vi "2D Histogram or PDF, PN.vi"(0 "Nbins U":i32, 1 "Nbins V":i32, 2 "Mean shift":bool, 3 "Umean":dbl, 4 "Vmean":dbl, 5 "Umax":dbl, 6 "No. of blocks":i32, 7 "Umin":dbl, 8 "PDF":bool, 9 "Interactive graph":bool, 10 "V":dbl[](array[numeric]), 11 "Vmax":dbl, 12 "U":dbl[](array[numeric]), 13 "Vmin":dbl) -> (14 "2D histogram or PDF":dbl[][](array[numeric]), 16 "U bin centre vals.":dbl[](array[numeric]), 17 "V bin centre vals.":dbl[](array[numeric]), 18 "UbinWidth":dbl, 19 "VbinWidth":dbl)   [LabVIEW 2011]
panel:
  in  "stop":bool
  in  "2D histogram or pdf":refnum<k7>(container)
  in  "show projections only":bool
  in  "yz projection":bool=TRUE
  in  "xz projection":bool=TRUE
  in  "xy projection":bool=TRUE
  in  "plot style":i32(ring)=9 items=["cwLine"=1, "cwPoint"=2, "cwLinePoint"=3, "cwHiddenLine"=4, "cwSurface"=5, "cwSurfaceLine"=6, "cwSurfaceNormal"=7, "cwContourLine"=8, "cwSurfaceContour"=9]
  in  "transparency":i32(knob)=40 scale=0.0..100.0
  # "N.B. The values of Umax, Umin, Vmax, Vmin, Umean, Vmean MUST be those of the ENTIRE dataset (i.e. all blocks) otherwise this routine will be inconsistent and therefore tell lies to you!!\n\nTo use this vi in a block by block manner, take note of the above and then simply add the resulting joint histogram / pdf array from each block as you go."
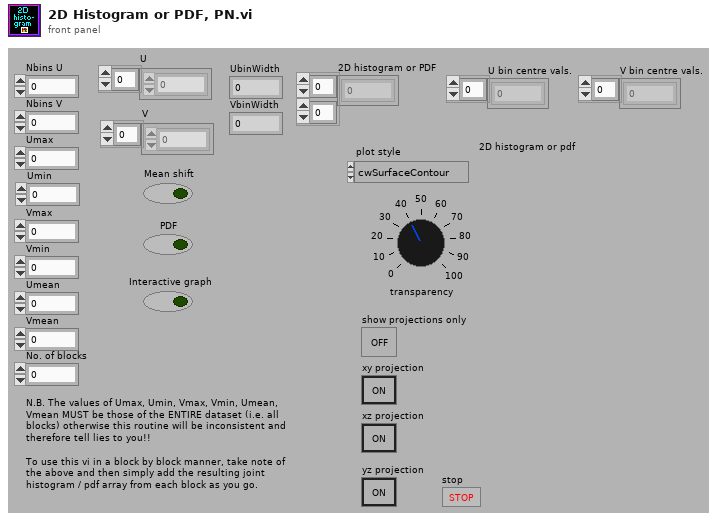
[diagram p1: front panel]
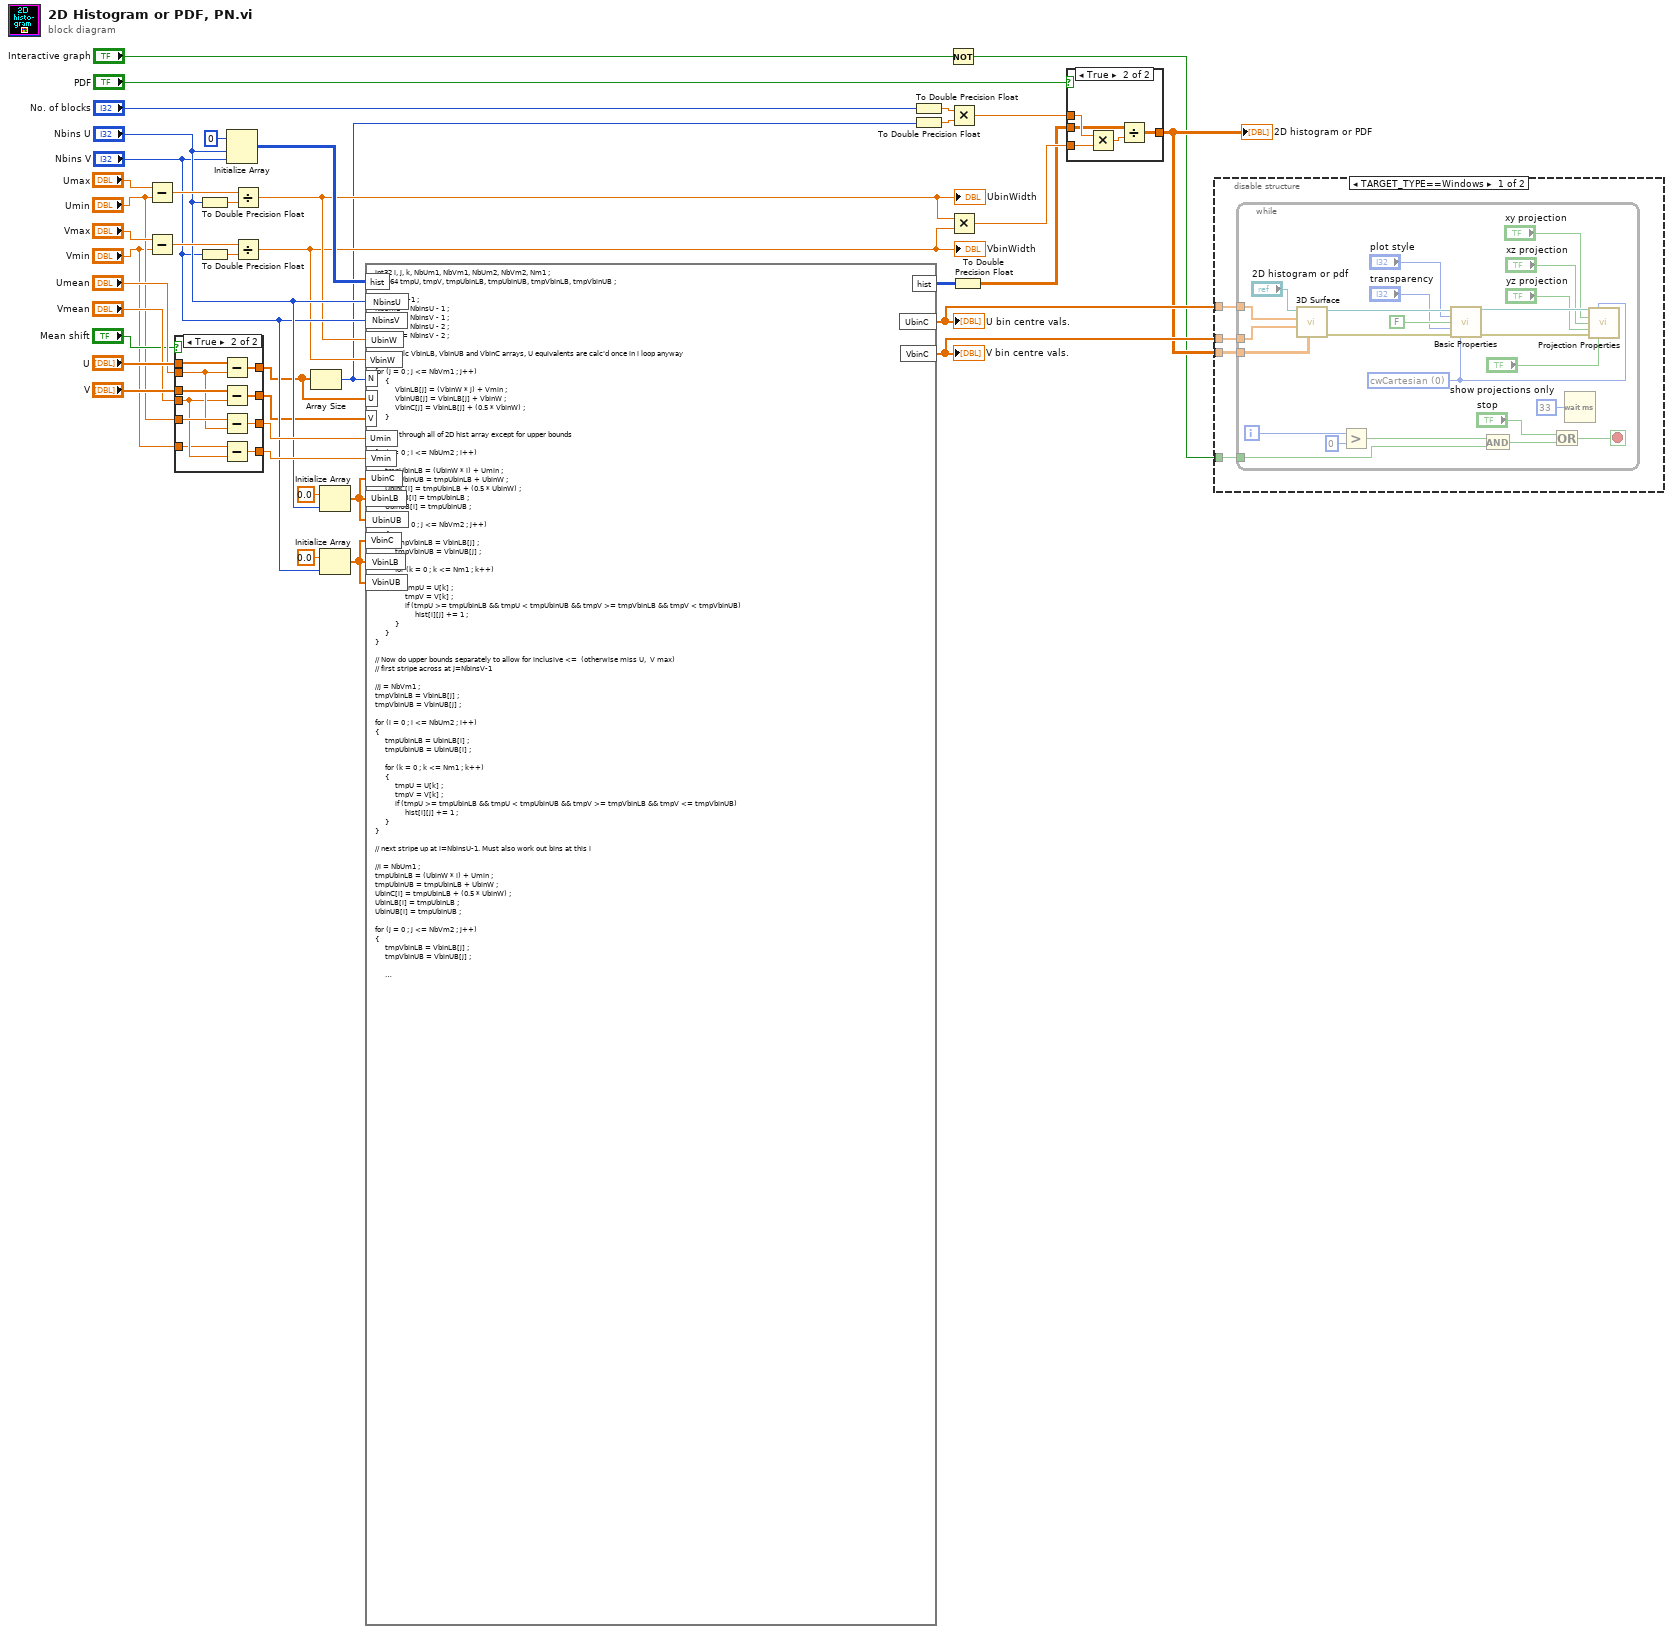
[diagram p0: block diagram]
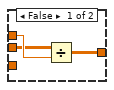
[diagram p3: hidden frame]
diagram:
  n1 = Subtract(x="Umax", y="Umin") -> (x-y=w28:dbl)
  n2 = Subtract(x="Vmax", y="Vmin") -> (x-y=w27:dbl)
  n3 = case shown="True" "Mean shift" {
    tunnel: "U" -> [w45 w55]
    tunnel: "V" -> [w44 w54]
    tunnel: "Vmean" -> [_ w49]
    tunnel: "Umean" -> [_ w50]
    tunnel: [w45 w53] -> w19
    tunnel: [w44 w52] -> w20
    tunnel: "Umin" -> [w43 w51]
    tunnel: "Vmin" -> [w42 w48]
    tunnel: [w42 w47] -> w25
    tunnel: [w43 w46] -> w26
    frame False {
    }
    frame True {
      n4 = Subtract(x=w55, y=w50) -> (x-y=w53:dbl[])
      n5 = Subtract(x=w54, y=w49) -> (x-y=w52:dbl[])
      n6 = Subtract(x=w51, y=w50) -> (x-y=w46:dbl)
      n7 = Subtract(x=w48, y=w49) -> (x-y=w47:dbl)
    }
  }
  n8 = To Double Precision Float(number="Nbins U") -> (double precision float=w41:dbl)
  n9 = To Double Precision Float(number="Nbins V") -> (double precision float=w40:dbl)
  n10 = Initialize Array(0 ("element"), "Nbins U", "Nbins V") -> (w33:i32[][])
  n11 = Divide(x=w28, y=w41) -> (x/y=w10:dbl)
  "UbinWidth" <- w10
  n12 = Divide(x=w27, y=w40) -> (x/y=w9:dbl)
  "VbinWidth" <- w9
  n13 = Array Size(array=w19) -> (size(s)=w1:i32)
  n14 = Initialize Array(0.0 ("element"), "Nbins U") -> (w18:dbl[])
  n15 = Initialize Array(0.0 ("element"), "Nbins V") -> (w17:dbl[])
  n16 = formula code="int32 i, j, k, NbUm1, NbVm1, NbUm2, NbVm2, Nm1 ;\nfloat64 tmpU, tmpV, tmpUbinLB, tmpUbinUB, tmpVbinLB, tmpVbinUB ;\n\nNm1 = N -1 ;\nNbUm1 = NbinsU - 1 ;\nNbVm1 = NbinsV - 1 ;\nNbUm2 = NbinsU - 2 ;\nNbVm2 = NbinsV - 2 ;\n\n// Pre-calc VbinLB, VbinUB and VbinC arrays, U equivalents are calc'd once in i loop anyway\n\nfor (j = 0 ; j <= NbVm1 ; j++)\n     {\n          VbinLB[j] = (VbinW * j) + Vmin ;\n          VbinUB[j] = VbinLB[j] + VbinW ;\n          VbinC[j] = VbinLB[j] + (0.5 * VbinW) ;\n     }\n\n// Loop through all of 2D hist array except for upper bounds\n\nfor (i = 0 ; i <= NbUm2 ; i++)\n{\n     tmpUbinLB = (UbinW * i) + Umin ;\n     tmpUbinUB = tmpUbinLB + UbinW ;\n     UbinC[i] = tmpUbinLB + (0.5 * UbinW) ;\n     UbinLB[i] = tmpUbinLB ;\n     UbinUB[i] = tmpUbinUB ;\n\n     for (j = 0 ; j <= NbVm2 ; j++)\n     {\n          tmpVbinLB = VbinLB[j] ;\n          tmpVbinUB = VbinUB[j] ;\n\n          for (k = 0 ; k <= Nm1 ; k++)\n          {\n               tmpU = U[k] ; \n               tmpV = V[k] ;\n               if (tmpU >= tmpUbinLB && tmpU < tmpUbinUB && tmpV >= tmpVbinLB && tmpV < tmpVbinUB)\n                    hist[i][j] += 1 ;\n          }\n     }          \n}\n\n// Now do upper bounds separately to allow for inclusive <=  (otherwise miss U,  V max)\n// first stripe across at j=NbinsV-1\n\n//j = NbVm1 ;\ntmpVbinLB = VbinLB[j] ;\ntmpVbinUB = VbinUB[j] ; \n\nfor (i = 0 ; i <= NbUm2 ; i++)\n{\n     tmpUbinLB = UbinLB[i] ;\n     tmpUbinUB = UbinUB[i] ;\n\n     for (k = 0 ; k <= Nm1 ; k++)\n     {\n          tmpU = U[k] ; \n          tmpV = V[k] ;\n          if (tmpU >= tmpUbinLB && tmpU < tmpUbinUB && tmpV >= tmpVbinLB && tmpV <= tmpVbinUB)\n               hist[i][j] += 1 ;\n     }        \n}\n\n// next stripe up at i=NbinsU-1. Must also work out bins at this i\n\n//i = NbUm1 ;\ntmpUbinLB = (UbinW * i) + Umin ;\ntmpUbinUB = tmpUbinLB + UbinW ;\nUbinC[i] = tmpUbinLB + (0.5 * UbinW) ;\nUbinLB[i] = tmpUbinLB ;\nUbinUB[i] = tmpUbinUB ;\n\nfor (j = 0 ; j <= NbVm2 ; j++)\n{\n     tmpVbinLB = VbinLB[j] ;\n     tmpVbinUB = VbinUB[j] ;\n\n     for (k = 0 ; k <= Nm1 ; k++)\n     {\n          tmpU = U[k] ; \n          tmpV = V[k] ;\n          if (tmpU >= tmpUbinLB && tmpU <= tmpUbinUB && tmpV >= tmpVbinLB && tmpV < tmpVbinUB)\n               hist[i][j] += 1 ;\n     }        \n}\n\n// Now finally do the last box in the top corner with both checks being <=\n\n//i = NbUm1 ;\n//j = NbVm1 ;\ntmpUbinLB = UbinLB[i] ;\ntmpUbinUB = UbinUB[i] ;\ntmpVbinLB = VbinLB[j] ;\ntmpVbinUB = VbinUB[j] ;\n\nfor (k = 0 ; k <= Nm1 ; k++)\n{\n     tmpU = U[k] ; \n     tmpV = V[k] ;\n     if (tmpU >= tmpUbinLB && tmpU <= tmpUbinUB && tmpV >= tmpVbinLB && tmpV <= tmpVbinUB)\n          hist[i][j] += 1 ;\n}"("NbinsU"="Nbins U", "NbinsV"="Nbins V", "N"=w1, "UbinW"=w10, "VbinW"=w9, "hist"=w33, "Umin"=w26, "Vmin"=w25, "UbinC"=w18, "VbinC"=w17, "U"=w19, "V"=w20, "UbinLB"=w18, "UbinUB"=w18, "VbinLB"=w17, "VbinUB"=w17) -> ("hist"=w7:i32[][], "UbinC"=w15:dbl[], "VbinC"=w16:dbl[])
  "U bin centre vals." <- w15
  "V bin centre vals." <- w16
  n17 = To Double Precision Float(number="No. of blocks") -> (double precision float=w12:dbl)
  n18 = To Double Precision Float(number=w1) -> (double precision float=w11:dbl)
  n19 = Not(x="Interactive graph") -> (.not. x?=w2:bool)
  n20 = Multiply(x=w12, y=w11) -> (x*y=w5:dbl)
  n21 = Multiply(x=w10, y=w9) -> (x*y=w8:dbl)
  n22 = To Double Precision Float(number=w7) -> (double precision float=w6:dbl[][])
  n23 = case shown="True" "PDF" {
    tunnel: w8 -> [_ w62]
    tunnel: w5 -> [w58 w63]
    tunnel: w6 -> [w57 w61]
    tunnel: [w56 w59] -> w4
    frame False {
      n24 = Divide(x=w57, y=w58) -> (x/y=w56:dbl[][])
    }
    frame True {
      n25 = Multiply(x=w63, y=w62) -> (x*y=w60:dbl)
      n26 = Divide(x=w61, y=w60) -> (x/y=w59:dbl[][])
    }
  }
  "2D histogram or PDF" <- w4
  n27 = disable-structure shown="TARGET_TYPE==Windows" {
    disable-tunnel: w16 -> [w67 _]
    disable-tunnel: w15 -> [w66 _]
    disable-tunnel: w4 -> [w65 _]
    disable-tunnel: w2 -> [w64 _]
    frame condition #0 {
      n28 = while {
        tunnel: w65 -> [w90]
        tunnel: w67 -> [w89]
        tunnel: w66 -> [w88]
        tunnel: w64 -> [w68]
        i -> [w74]
        stop <- w72 stop-if-true
        w82 = 0 items=["cwCartesian", "cwCylindrical", "cwSpherical"] ("coordinate system")
        n29 = call <vilib>:"3D Surface.vi"("z matrix"=w90, "y vector"=w89, "x vector"=w88, "3D graph"="2D histogram or pdf") -> ("error out"=w86:errorcluster, "3D graph out"=w87:refnum<k7>)  [unwired: 6 in]
        n30 = Greater?(x=w74, y=0) -> (0:w69:bool)
        n31 = call <vilib>:"Basic Properties.vi"("3D graph"=w87, "plot style"="plot style", "fast draw"=FALSE, "transparency"="transparency", "error in (no error)"=w86, "coordinate system"=w82) -> ("3D graph out"=w85:refnum<k7>, "error out"=w84:errorcluster)  [unwired: 8 in]
        n32 = And(x=w69, y=w68) -> (x .and. y?=w70:bool)
        n33 = Or(x="stop", y=w70) -> (x .or. y?=w72:bool)
        n34 = Wait (ms)(milliseconds to wait=u32 33) -> ()  [unwired: 1 out]
        n35 = call <vilib>:"Projection Properties.vi"("3D graph"=w85, "coordinate system"=w82, "xy projection"="xy projection", "xz projection"="xz projection", "yz projection"="yz projection", "error in (no error)"=w84, "show projections only"="show projections only") -> ()  [unwired: 7 in, 2 out]
      }
    }
    frame condition #1 (active) {
    }
  }
